vi "超标留样启动.vi"(8 "error in (no error)":errorcluster) -> (0 "error out":errorcluster)   [LabVIEW 2016, in "德润超标留样.lvlib"]
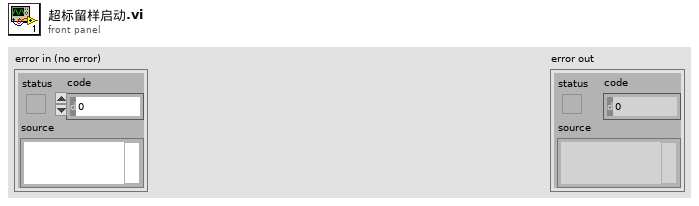
[diagram p1: front panel]
types:
  T1 = enum16{"open", "read", "write", "write single", "close"}
  T2 = cluster{"STEP":enum16{"open", "read", "write", "write single", "close"}, "starting address":u16, "value":u16}
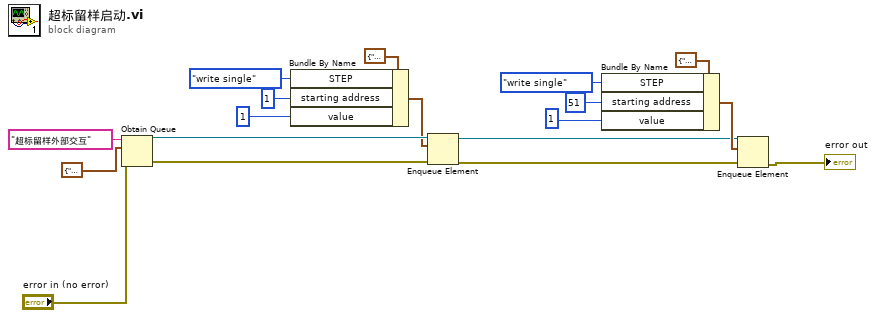
[diagram p0: block diagram]
diagram:
  n1 = Obtain Queue(name (unnamed)="超标留样外部交互" ("名称（未命名）"), element data type=T2 {"STEP"=enum."write single", "starting address"=0, "value"=0}, error in (no error)="error in (no error)") -> (queue out=w5:refnum<queue>, error out=w3:errorcluster)  [unwired: 2 in, 1 out]
  n2 = Bundle By Name(cluster=T2 {"STEP"=enum."open", "starting address"=0, "value"=0} ("元素"), "STEP"=T1."write single", "starting address"=u16 1, "value"=u16 1) -> (w4:T2)
  n3 = Enqueue Element(queue=w5, element=w4, error in (no error)=w3) -> (queue out=w2:refnum<queue>, error out=w1:errorcluster)  [unwired: 1 in, 1 out]
  n4 = Bundle By Name(cluster=T2 {"STEP"=enum."open", "starting address"=0, "value"=0} ("元素"), "STEP"=T1."write single", "starting address"=u16 51, "value"=u16 1) -> (w15:T2)
  n5 = Enqueue Element(queue=w2, element=w15, error in (no error)=w1) -> (error out=→"error out":errorcluster)  [unwired: 1 in, 2 out]
